vi "resample_test.vi"() -> ()   [LabVIEW 2024]
uses:
  Vision.lvlib
panel:
  in  "height":i32=40
  in  "width":i32=20
  in  "File Path":path=path "C:/Users/Caleb/Desktop/obama.jpg"
  out "error out":errorcluster
  out "Image":T1(plugin-control)
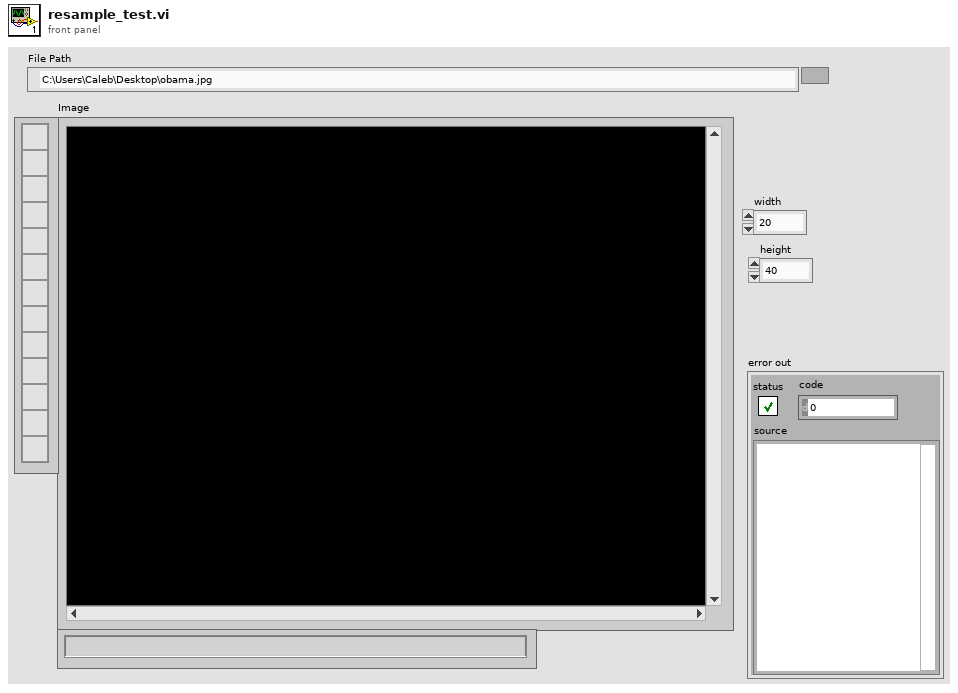
[diagram p1: front panel]
types:
  T1 = typedef "IMAQ Image.ctl" = refnum<image>
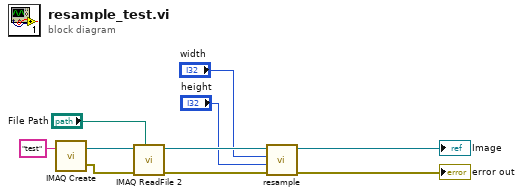
[diagram p0: block diagram]
diagram:
  n1 = call "IMAQ Create"("Image Name"="test") -> ("New Image"=w10:T1, "error out"=w8:errorcluster)  [unwired: 4 in]
  n2 = call "IMAQ ReadFile 2"("File Path"="File Path", "error in (no error)"=w8, "Image"=w10) -> ("error out"=w3:errorcluster, "Image Out"=w6:T1)  [unwired: 4 in, 3 out]
  n3 = call "resample.vi"("error in (no error)"=w3, "Height"="height", "Width"="width", "Image in"=w6) -> ("error out"=→"error out":errorcluster, "Image out"=→"Image":T1)  [unwired: 6 in]
